vi "main.vi"   [LabVIEW 2020]
uses:
  <userlib>/_NEVSTOP/GlobalStop/_gStop.vi
  <userlib>/_NEVSTOP/GlobalStop/GSTOP.lvlib
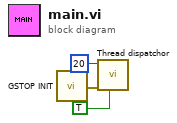
[diagram p0: block diagram]
diagram:
  n1 = call <userlib>:"GSTOP INIT.vi"() -> ("error out"=w1:errorcluster)  [unwired: 15 in]
  n2 = call "Thread dispatchor.vi"("open fp?"=TRUE, "error in (no error)"=w1, "Numeric"=20) -> ()  [unwired: 8 in, 1 out]
